vi "校准任务流程.vi"(9 "校准任务":T1[](array[typedef]), 10 "精度":dbl=4.0, 11 "模型":enum32{"线性", "多项式", "折线"}(ring)) -> ()   [LabVIEW 2016]
uses:
  <userlib>/_OpenG.lib/array/array.llb/Remove Duplicates from 1D Array (U16)__ogtk.vi
panel:
  out "元素":T1
  out "执行列表":T2(ring)
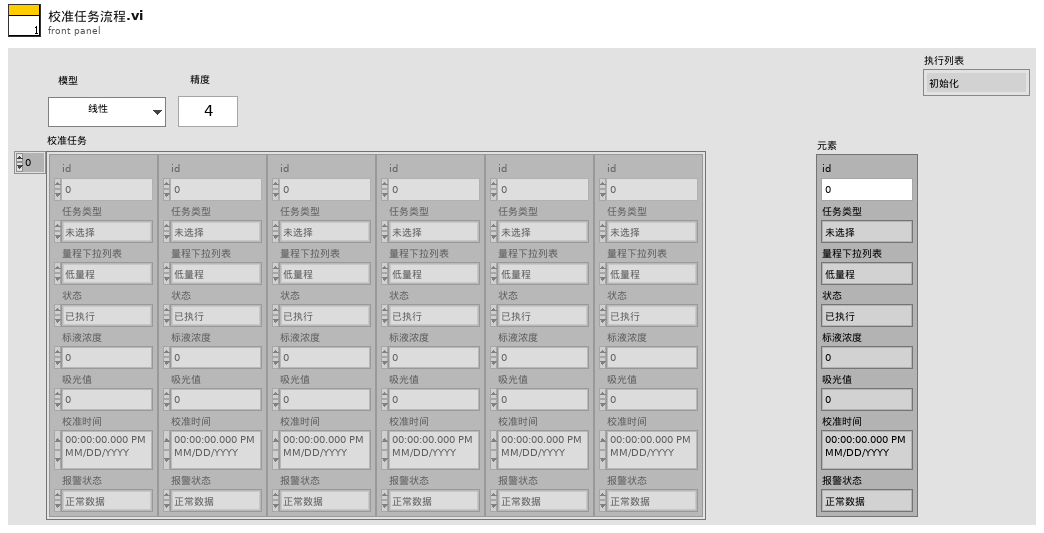
[diagram p1: front panel]
types:
  T1 = typedef "校准任务.ctl" = cluster{"id":u16, "任务类型":enum16{"未选择", "空白校准", "标样校准", "标样核查", "零点核查", "跨度核查"}, "量程下拉列表":enum16{"低量程", "高量程"}, "状态":enum16{"已执行", "待执行", "执行中", "停止"}, "标液浓度":dbl, "吸光值":dbl, "校准时间":timestamp, "报警状态":enum16{"正常数据", "报警数据"}}
  T2 = enum16{"初始化", "解析数据", "判断任务类型", "执行测试任务", "等待测试任务完成", "获取测试数据", "任务结束判定", "计算公式", "结束"}
  T3 = cluster{"时间标识":timestamp, "设备":string, "日志信息":string, "流程参数":string}
  T4 = cluster{"站号":u16, "量程切换":enum32{"H", "L", "AUTO"}, "控制命令":u16, "模式设置":enum16{"待机", "连续模式", "周期模式", "定点模式", "受控模式", "手动模式"}, "测量间隔":u16}
  T5 = cluster{"标液浓度1":dbl, "测量吸光度1":dbl, "样品1启用":bool, "标液浓度2":dbl, "测量吸光度2":dbl, "样品2启用":bool, "标液浓度3":dbl, "测量吸光度3":dbl, "样品3启用":bool, "标液浓度4":dbl, "测量吸光度4":dbl, "样品4启用":bool, "标液浓度5":dbl, "测量吸光度5":dbl, "样品5启用":bool, "模型":enum32{"线性", "多项式", "折线"}, "精度":dbl, "XY图":cluster{"X Values":dbl[], "Y Values":dbl[]}[], "拟合公式":string, "r^2":dbl, "标样一校准时间":timestamp, "标样二校准时间":timestamp, "标样三校准时间":timestamp, "标样四校准时间":timestamp, "标样五校准时间":timestamp, "二次方程":cluster{"x^2":dbl, "K":dbl, "B":dbl}, "标定时间":timestamp, "拟合公式 2":string, "r^2 2":dbl}
  T6 = enum16{"", "水样测量", "标样核查", "零点核查", "跨度核查", "空白测试", "平行样测试", "加标回收", "空白校准", "标样校准"}
  T7 = typedef "报警信息字段定义.ctl" = cluster{"时间":timestamp, "参数":string, "元器件":string, "故障现象":string, "故障分析":string, "state":string, "code":string, "platform_alarm_code":string}
  T8 = cluster{"测量精度":u16, "消解温度":u16, "消解时长":u16, "量程下限":sgl, "量程上限":sgl, "曲线斜率K":sgl, "曲线斜率B":sgl, "标定日期":timestamp, "标液1浓度":sgl, "标液1测量过程值":sgl, "标液2浓度":sgl, "标液2测量过程值":sgl, "标液3浓度":sgl, "标液3测量过程值":sgl, "标液4浓度":sgl, "标液4测量过程值":sgl, "标液5浓度":sgl, "标液5测量过程值":sgl, "线性相关系数":sgl, "试剂余量":u32, "测量滴定值或吸光度":sgl, "标样2校准时间":timestamp, "检出限值":sgl, "校准系数":sgl, "设备系列号":string, "显色温度":u16, "显色时间":u16, "试剂余量1":u16, "试剂余量2":u16, "试剂余量3":u16, "试剂余量4":u16, "试剂余量5":u16, "试剂余量6":u16, "试剂余量7":u16, "试剂余量8":u16, "试剂余量9":u16, "试剂余量10":u16, "当前量程低位":sgl, "当前量程高位":sgl}
  T9 = cluster{"因子编码":u32, "单位":u16, "标样2参考值":sgl, "水样数据时间":timestamp, "水样实测值":sgl, "水样数据标识":string, "标样2数据时间":timestamp, "标样2实测值":sgl, "标样2数据标识":string, "空白数据时间":timestamp, "空白实测值":sgl, "空白数据标识":string, "零点核查数据时间":timestamp, "零点核查实测值":sgl, "零点核查数据标识":string, "跨度核查数据时间":timestamp, "跨度核查实测值":sgl, "跨度核查数据标识":string, "加标回收数据时间":timestamp, "加标回收实测值":sgl, "加标回收数据标识":string, "平行样数据时间":timestamp, "平行样实测值":sgl, "平行样数据标识":string, "标样1参考值":sgl, "标样1数据时间":timestamp, "标样1实测值":sgl, "标样1数据标识":string, "标样核查数据时间":timestamp, "标样核查实测值":sgl, "标样核查数据标识":string}
  T10 = cluster{"系统时间":timestamp, "工作状态":u16, "测量模式":enum16{"待机", "连续模式", "周期模式", "定点模式", "受控模式", "手动模式"}, "告警代码":u16, "故障代码":u16, "日志代码":u16, "软件版本":u16, "测量间隔":u16, "消解实时温度":dbl, "校准间隔（天）":u16, "校准间隔（时）":u16, "周期测量时间（23_16）":u16, "周期测量时间（15_0）":u16, "清洗周期（次数）":u16, "运行模式":u16, "自动校准状态":u16, "自动清洗状态":u16}
  T11 = enum16{"未选择", "空白校准", "标样校准", "标样核查", "零点核查", "跨度核查"}
  T12 = cluster{"标液浓度1":dbl, "测量吸光度1":dbl, "样品1启用":bool, "标液浓度2":dbl, "测量吸光度2":dbl, "样品2启用":bool, "标液浓度3":dbl, "测量吸光度3":dbl, "样品3启用":bool, "标液浓度4":dbl, "测量吸光度4":dbl, "样品4启用":bool, "标液浓度5":dbl, "测量吸光度5":dbl, "样品5启用":bool, "模型":enum32{"线性", "多项式", "折线"}, "精度":dbl, "XY图":cluster{"X Values":dbl[], "Y Values":dbl[]}[], "拟合公式":string, "r^2":dbl, "标样一校准时间":timestamp, "标样二校准时间":timestamp, "标样三校准时间":timestamp, "标样四校准时间":timestamp, "标样五校准时间":timestamp, "二次方程":cluster{"c":dbl, "x":dbl, "x^2":dbl}, "标定时间":timestamp, "拟合公式 2":string, "r^2 2":dbl}
  T13 = cluster{"标液浓度1":dbl, "测量吸光度1":dbl, "样品1启用":bool, "标液浓度2":dbl, "测量吸光度2":dbl, "样品2启用":bool, "标液浓度3":dbl, "测量吸光度3":dbl, "样品3启用":bool, "标液浓度4":dbl, "测量吸光度4":dbl, "样品4启用":bool, "标液浓度5":dbl, "测量吸光度5":dbl, "样品5启用":bool, "模型":enum32{"线性", "多项式", "折线"}, "精度":dbl, "XY图":cluster{"X Values":dbl[], "Y Values":dbl[]}[], "拟合公式":string, "r^2":dbl, "标样一校准时间":timestamp, "标样二校准时间":timestamp, "标样三校准时间":timestamp, "标样四校准时间":timestamp, "标样五校准时间":timestamp, "二次方程":cluster{"c":dbl, "x":dbl, "x^2":dbl}, "标定时间":timestamp, "拟合公式 2":string, "r^2 2":dbl}[][]
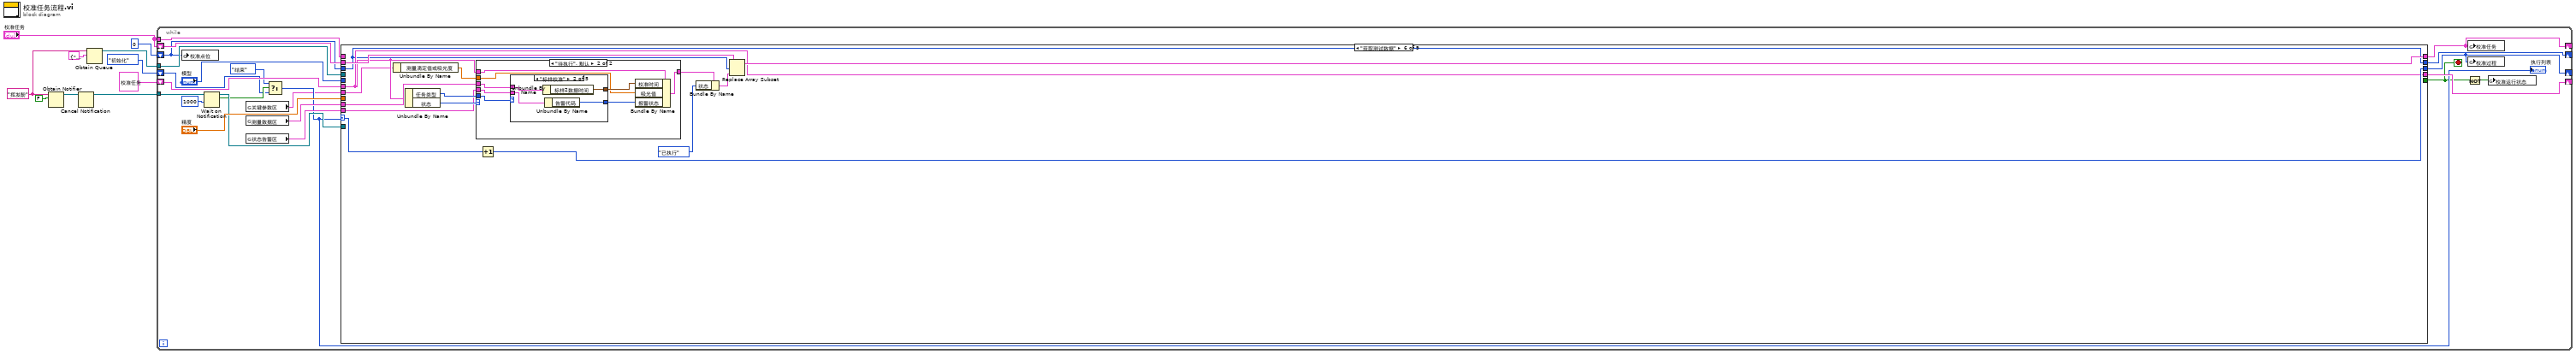
[diagram p0: block diagram]
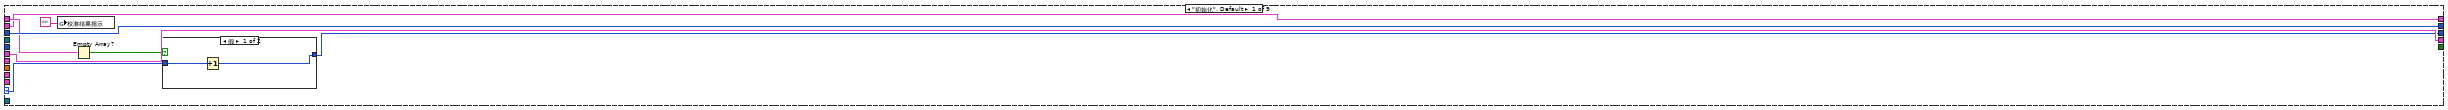
[diagram p2: hidden frame]
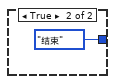
[diagram p3: hidden frame]
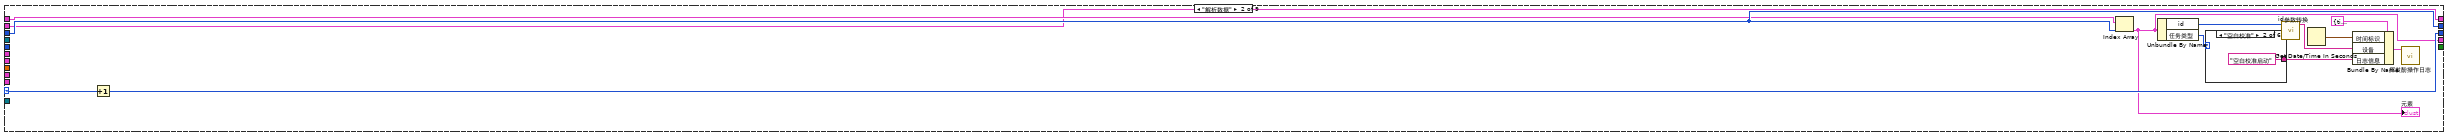
[diagram p4: hidden frame]
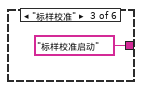
[diagram p6: hidden frame]
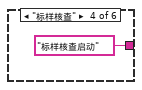
[diagram p7: hidden frame]
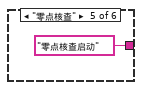
[diagram p8: hidden frame]
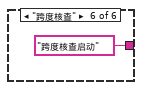
[diagram p9: hidden frame]
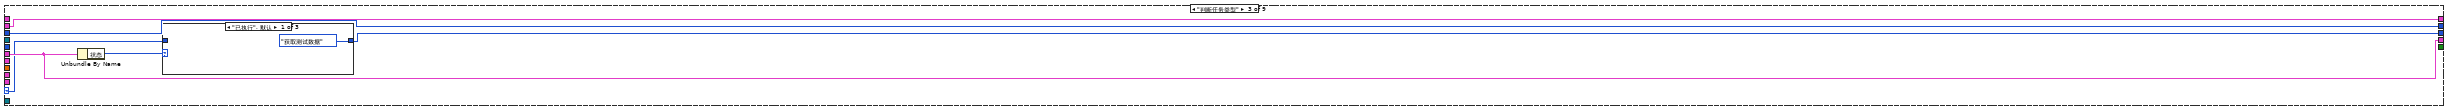
[diagram p10: hidden frame]
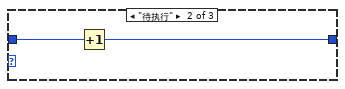
[diagram p11: hidden frame]
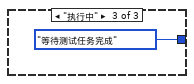
[diagram p12: hidden frame]
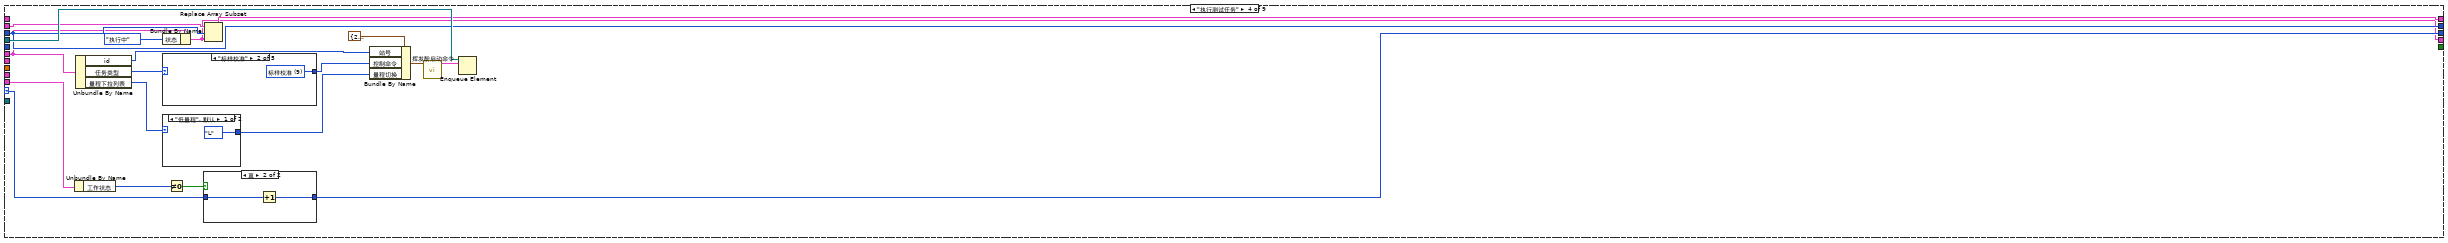
[diagram p13: hidden frame]
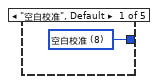
[diagram p15: hidden frame]
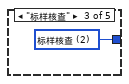
[diagram p16: hidden frame]
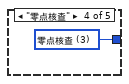
[diagram p17: hidden frame]
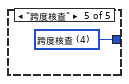
[diagram p18: hidden frame]
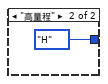
[diagram p19: hidden frame]
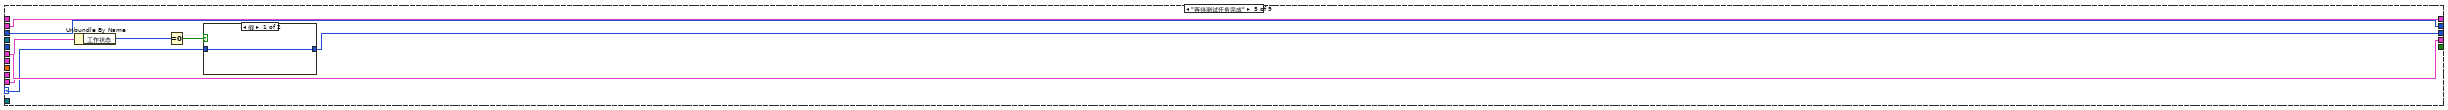
[diagram p20: hidden frame]
diagram:
  w2 = "挥发酚" ("名称（未命名）")
  n1 = Obtain Notifier(name (unnamed)=w2, notification data type=FALSE) -> (notifier out=w5:refnum<notifier>)  [unwired: 2 in, 2 out]
  n2 = Cancel Notification(0:w5) -> (8:w4:refnum<notifier>)  [unwired: 1 in, 2 out]
  n3 = Obtain Queue(name (unnamed)=w2, element data type=cluster{"命令":string, "data":variant} {"命令"="", "data"=variant}) -> (queue out=w6:refnum<queue>)  [unwired: 3 in, 2 out]
  n4 = while {
    shift-right: [w13] -> _
    shift-left: 0 -> [w15]
    shift-right: [w33] -> _
    shift-left: T1 {"id"=0, "任务类型"=enum."未选择", "量程下拉列表"=enum."低量程", "状态"=enum."待执行", "标液浓度"=0.0, "吸光值"=0.0, "校准时间"=timestamp(0 s since 1904-01-01), "报警状态"=enum."正常数据"} ("校准任务") -> [w32]
    shift-right: [w12] -> _
    shift-left: T2."初始化" ("执行列表") -> [w21]
    tunnel: w6 -> [w31]
    tunnel: w4 -> [w30]
    tunnel: "校准任务" -> [w27]
    shift-right: [w14] -> _
    shift-left: "校准任务" -> [w26]
    stop <- w16 stop-if-true
    n5 = global write "VAR挥发酚全局变量.vi" "校准点位"(w15) -> ()
    n6 = Wait on Notification(notifier=w30, timeout in ms (-1)=1000 ("超时毫秒(-1)")) -> (notifier out=w23:refnum<notifier>, notification=w22:bool)  [unwired: 2 in, 2 out]
    n7 = global read "VAR挥发酚全局变量.vi" "关键参数区"() -> (w11:T8)
    n8 = global read "VAR挥发酚全局变量.vi" "测量数据区"() -> (w28:T9)
    n9 = global read "VAR挥发酚全局变量.vi" "状态告警区"() -> (w29:T10)
    n10 = Select(t=T2."结束", s=w22, f=w21) -> (s? t:f=w20:T2)
    "执行列表" <- w20
    n11 = case shown="\"获取测试数据\"" w20 {
      selector: w20 -> [w39 w56 w65 w83 w106 w126 w164 w178 w372]
      tunnel: w15 -> [w40 w57 w67 w79 w109 w117 w165 w176 w370]
      tunnel: [w41 w48 w68 w76 w110 w121 w166 w175 w371] -> w33
      tunnel: w32 -> [w41 _ w68 w78 w110 w121 w166 w175 w371]
      tunnel: [w40 w57 w67 w79 w109 w117 w161 w176 w370] -> w13
      tunnel: [_ _ _ _ _ _ _ _ TRUE] -> w16
      tunnel: [w38 w55 w64 w82 w104 w125 w163 w177 w372] -> w12
      tunnel: w31 -> [_ _ _ w91 _ _ _ _ w367]
      tunnel: w23 -> [_ _ _ _ _ _ _ _ w366]
      tunnel: w29 -> [_ _ _ w86 w108 w116 _ _ _]
      tunnel: w28 -> [_ _ _ _ _ w128 _ _ _]
      tunnel: w27 -> [w36 w54 _ _ _ _ w162 _ _]
      tunnel: [w35 w53 w63 w80 w103 w123 w158 w174 w368] -> w14
      tunnel: w26 -> [w35 w53 w63 w81 w103 w122 w158 w174 w368]
      tunnel: "模型" -> [_ _ _ _ _ _ _ w173 _]
      tunnel: "精度" -> [_ _ _ _ _ _ _ w172 _]
      tunnel: w11 -> [_ _ _ _ _ w115 _ _ _]
      frame "初始化", Default {
        n12 = global write "VAR挥发酚全局变量.vi" "校准结果指示"("") -> ()
        n13 = Empty Array?(array=w36) -> (empty?=w34:bool)
        n14 = case shown="假" w34 {
          tunnel: w39 -> [w43 _]
          tunnel: [w42 T2."结束"] -> w38
          frame False {
            n15 = Increment(x=w43) -> (x+1=w42:T2)
          }
          frame True {
          }
        }
      }
      frame "解析数据" {
        n16 = Increment(x=w56) -> (x+1=w55:T2)
        n17 = Index Array(array=w54, index=w57) -> (element=w48:T1)
        "元素" <- w48
        n18 = Unbundle By Name(w48) -> ("id"=w47:u16, "任务类型"=w46:T11)
        n19 = case shown="\"空白校准\"" w46 {
          tunnel: [_ "空白校准启动" "标样校准启动" "标样核查启动" "零点核查启动" "跨度核查启动"] -> w45
          frame "未选择", Default {
          }
          frame "空白校准" {
          }
          frame "标样校准" {
          }
          frame "标样核查" {
          }
          frame "零点核查" {
          }
          frame "跨度核查" {
          }
        }
        n20 = call "id参数转换.vi"("id"=w47) -> ("table输出"=w49:string)  [unwired: 10 in]
        n21 = Get Date/Time In Seconds() -> (seconds since 1Jan1904=w52:timestamp)
        n22 = Bundle By Name(cluster=T3 {"时间标识"=timestamp(0 s since 1904-01-01), "设备"="", "日志信息"="", "流程参数"=""} ("data in"), "时间标识"=w52, "设备"=w49, "日志信息"=w45) -> (w51:T3)
        n23 = call "挥发酚操作日志.vi"("data in"=w51) -> ()  [unwired: 11 in]
      }
      frame "判断任务类型" {
        n24 = Unbundle By Name(w68) -> ("状态"=w66:enum16{"已执行", "待执行", "执行中", "停止"})
        n25 = case shown="\"已执行\", 默认" w66 {
          tunnel: w65 -> [_ w71 _]
          tunnel: [T2."获取测试数据" w70 T2."等待测试任务完成"] -> w64
          frame "已执行", Default {
          }
          frame "待执行" {
            n26 = Increment(x=w71) -> (x+1=w70:T2)
          }
          frame "执行中" {
          }
        }
      }
      frame "执行测试任务" {
        n27 = Unbundle By Name(w86) -> ("工作状态"=w85:u16)
        n28 = Unbundle By Name(w78) -> ("id"=w90:u16, "任务类型"=w89:T11, "量程下拉列表"=w88:enum16{"低量程", "高量程"})
        n29 = Bundle By Name(cluster=w78, "状态"=enum16{"已执行", "待执行", "执行中", "停止"}."执行中") -> (w76:T1)
        n30 = case shown="\"标样校准\"" w89 {
          tunnel: [w96 w97 w98 w99 w100] -> w73
          frame "空白校准", Default {
            w96 = u16 8 items=["启动测量"=1, "标样核查"=2, "零点核查"=3, "跨度核查"=4, "空白测试"=5, "平行样测试"=6, "加标回收"=7, "空白校准"=8, "标样校准"=9, "初始化（清洗）"=10, "停止测试"=11, "仪器重启"=12, "校时"=13, "模式设置"=14, "测量间隔设置"=15, "调试"=22, "填充管路"=30, "清洗管路"=31, "清洗反应杯"=32] ("控制命令")
          }
          frame "标样校准" {
            w97 = u16 9 items=["启动测量"=1, "标样核查"=2, "零点核查"=3, "跨度核查"=4, "空白测试"=5, "平行样测试"=6, "加标回收"=7, "空白校准"=8, "标样校准"=9, "初始化（清洗）"=10, "停止测试"=11, "仪器重启"=12, "校时"=13, "模式设置"=14, "测量间隔设置"=15, "调试"=22, "填充管路"=30, "清洗管路"=31, "清洗反应杯"=32] ("控制命令")
          }
          frame "标样核查" {
            w98 = u16 2 items=["启动测量"=1, "标样核查"=2, "零点核查"=3, "跨度核查"=4, "空白测试"=5, "平行样测试"=6, "加标回收"=7, "空白校准"=8, "标样校准"=9, "初始化（清洗）"=10, "停止测试"=11, "仪器重启"=12, "校时"=13, "模式设置"=14, "测量间隔设置"=15, "调试"=22, "填充管路"=30, "清洗管路"=31, "清洗反应杯"=32] ("控制命令")
          }
          frame "零点核查" {
            w99 = u16 3 items=["启动测量"=1, "标样核查"=2, "零点核查"=3, "跨度核查"=4, "空白测试"=5, "平行样测试"=6, "加标回收"=7, "空白校准"=8, "标样校准"=9, "初始化（清洗）"=10, "停止测试"=11, "仪器重启"=12, "校时"=13, "模式设置"=14, "测量间隔设置"=15, "调试"=22, "填充管路"=30, "清洗管路"=31, "清洗反应杯"=32] ("控制命令")
          }
          frame "跨度核查" {
            w100 = u16 4 items=["启动测量"=1, "标样核查"=2, "零点核查"=3, "跨度核查"=4, "空白测试"=5, "平行样测试"=6, "加标回收"=7, "空白校准"=8, "标样校准"=9, "初始化（清洗）"=10, "停止测试"=11, "仪器重启"=12, "校时"=13, "模式设置"=14, "测量间隔设置"=15, "调试"=22, "填充管路"=30, "清洗管路"=31, "清洗反应杯"=32] ("控制命令")
          }
        }
        n31 = case shown="\"低量程\", 默认" w88 {
          tunnel: [enum32{"H", "L", "AUTO"}."L" ("量程切换") enum32{"H", "L", "AUTO"}."H" ("量程切换")] -> w87
          frame "低量程", Default {
          }
          frame "高量程" {
          }
        }
        n32 = Not Equal To 0?(x=w85) -> (x != 0?=w84:bool)
        n33 = case shown="真" w84 {
          tunnel: w83 -> [w93 w95]
          tunnel: [w93 w94] -> w82
          frame False {
          }
          frame True {
            n34 = Increment(x=w95) -> (x+1=w94:T2)
          }
        }
        n35 = Replace Array Subset(array=w81, new element=w76, index=w79) -> (w80:T1[])
        n36 = Bundle By Name(cluster=T4 {"站号"=21, "量程切换"=enum."AUTO", "控制命令"=0, "模式设置"=enum."待机", "测量间隔"=0} ("参数"), "站号"=w90, "控制命令"=w73, "量程切换"=w87) -> (w74:T4)
        n37 = call "挥发酚启动命令.vi"("参数"=w74) -> ("启动命令"=w92:cluster{"命令":string, "data":variant})  [unwired: 10 in]
        n38 = Enqueue Element(queue=w91, element=w92) -> ()  [unwired: 2 in, 3 out]
      }
      frame "等待测试任务完成" {
        n39 = Unbundle By Name(w108) -> ("工作状态"=w107:u16)
        n40 = Equal To 0?(x=w107) -> (x = 0?=w105:bool)
        n41 = case shown="假" w105 {
          tunnel: w106 -> [w111 w113]
          tunnel: [w111 w112] -> w104
          frame False {
          }
          frame True {
            n42 = Increment(x=w113) -> (x+1=w112:T2)
          }
        }
      }
      frame "获取测试数据" {
        n43 = Unbundle By Name(w115) -> ("测量滴定值或吸光度"=w114:sgl)
        n44 = Unbundle By Name(w121) -> ("任务类型"=w127:T11, "状态"=w120:enum16{"已执行", "待执行", "执行中", "停止"})
        n45 = case shown="\"待执行\", 默认" w120 {
          tunnel: w128 -> [_ w137]
          tunnel: w127 -> [_ w136]
          tunnel: [w129 w134] -> w124
          tunnel: w121 -> [w129 w133]
          tunnel: w116 -> [_ w132]
          tunnel: w114 -> [_ w130]
          frame "已执行" {
          }
          frame "待执行", Default {
            n46 = case shown="\"标样校准\"" w136 {
              tunnel: w137 -> [w141 w145 w149 w153 w157]
              tunnel: [w140 w144 w148 w152 w156] -> w135
              tunnel: w132 -> [w139 w143 w147 w151 w155]
              tunnel: [w138 w142 w146 w150 w154] -> w131
              frame "空白校准", Default {
                n47 = Unbundle By Name(w141) -> ("空白数据时间"=w140:timestamp)
                n48 = Unbundle By Name(w139) -> ("告警代码"=w138:u16)
              }
              frame "标样校准" {
                n49 = Unbundle By Name(w145) -> ("标样2数据时间"=w144:timestamp)
                n50 = Unbundle By Name(w143) -> ("告警代码"=w142:u16)
              }
              frame "标样核查" {
                n51 = Unbundle By Name(w149) -> ("标样2数据时间"=w148:timestamp)
                n52 = Unbundle By Name(w147) -> ("告警代码"=w146:u16)
              }
              frame "零点核查" {
                n53 = Unbundle By Name(w153) -> ("零点核查数据时间"=w152:timestamp)
                n54 = Unbundle By Name(w151) -> ("告警代码"=w150:u16)
              }
              frame "跨度核查" {
                n55 = Unbundle By Name(w157) -> ("跨度核查数据时间"=w156:timestamp)
                n56 = Unbundle By Name(w155) -> ("告警代码"=w154:u16)
              }
            }
            n57 = Bundle By Name(cluster=w133, "校准时间"=w135, "吸光值"=w130, "报警状态"=w131) -> (w134:T1)
          }
        }
        n58 = Increment(x=w126) -> (x+1=w125:T2)
        n59 = Bundle By Name(cluster=w124, "状态"=enum16{"已执行", "待执行", "执行中", "停止"}."已执行") -> (w118:T1)
        n60 = Replace Array Subset(array=w122, new element=w118, index=w117) -> (w123:T1[])
      }
      frame "任务结束判定" {
        n61 = Array Size(array=w162) -> (size(s)=w160:i32)
        n62 = Increment(x=w165) -> (x+1=w161:i32)
        n63 = Greater Or Equal?(x=w161, y=w160) -> (x >= y?=w159:bool)
        n64 = case shown="假" w159 {
          tunnel: w164 -> [_ w170]
          tunnel: [T2."解析数据" w169] -> w163
          frame False {
            n65 = Wait (ms)(milliseconds to wait=u32 3000 ("等待时间（毫秒）")) -> ()  [unwired: 1 out]
          }
          frame True {
            n66 = Increment(x=w170) -> (x+1=w169:T2)
          }
        }
      }
      frame "计算公式" {
        n67 = flat-sequence {
          tunnel: w178 -> [w185]
          tunnel: w174 -> [w181]
          tunnel: w173 -> [w180]
          tunnel: w172 -> [w179]
          tunnel: [w184] -> w171
          tunnel: [w365] -> w177
          tunnel: w171 -> [w365]
          frame #0 {
            n68 = for {
              tunnel: w181 -> [w364] mode=indexing
              tunnel: [w363] -> w183 mode=indexing
              n69 = Unbundle By Name(w364) -> ("id"=w363:u16)
            }
            n70 = Increment(x=w185) -> (x+1=w184:T2)
            n71 = call-poly <userlib>:"Remove Duplicates from 1D Array__ogtk.vi"("Input Array"=w183) -> ("Output Array"=w182:u16[])  [unwired: 1 out]
            n72 = for {
              tunnel: w182 -> [w198] mode=indexing
              tunnel: w181 -> [w200]
              tunnel: w180 -> [w197]
              tunnel: w179 -> [w196]
              n73 = for {
                tunnel: w200 -> [w360] mode=indexing
                tunnel: w198 -> [w362]
                tunnel: [w360] -> w199 mode=indexing if=w361
                n74 = Unbundle By Name(w360) -> ("id"=w359:u16)
                n75 = Equal?(x=w359, y=w362) -> (x = y?=w361:bool)
              }
              n76 = flat-sequence {
                tunnel: w199 -> [w213]
                tunnel: w198 -> [w208]
                tunnel: w197 -> [w212]
                tunnel: w196 -> [w211]
                tunnel: T5 {"标液浓度1"=0.0, "测量吸光度1"=0.0, "样品1启用"=FALSE, "标液浓度2"=0.0, "测量吸光度2"=0.0, "样品2启用"=FALSE, "标液浓度3"=0.0, "测量吸光度3"=0.0, "样品3启用"=FALSE, "标液浓度4"=0.0, "测量吸光度4"=0.0, "样品4启用"=FALSE, "标液浓度5"=0.0, "测量吸光度5"=0.0, "样品5启用"=FALSE, "模型"=enum."线性", "精度"=4.0, "XY图"=[], "拟合公式"="", "r^2"=0.0, "标样一校准时间"=timestamp(0 s since 1904-01-01), "标样二校准时间"=timestamp(0 s since 1904-01-01), "标样三校准时间"=timestamp(0 s since 1904-01-01), "标样四校准时间"=timestamp(0 s since 1904-01-01), "标样五校准时间"=timestamp(0 s since 1904-01-01), "二次方程"={"x^2"=0.0, "K"=0.0, "B"=0.0}, "标定时间"=timestamp(0 s since 1904-01-01), "拟合公式 2"="", "r^2 2"=0.0} ("曲线模型") -> [w210]
                tunnel: [w209] -> w195
                tunnel: [w208] -> w194
                tunnel: [w207] -> w193
                tunnel: [w206] -> w191
                tunnel: cluster{"x^2":dbl, "K":dbl, "B":dbl} {"x^2"=0.0, "K"=0.0, "B"=0.0} ("二次方程 2") -> [w205]
                tunnel: [w204] -> w190
                tunnel: 0.0 ("公式切换阈值滴定数(0~9999)") -> [w203]
                tunnel: [w202] -> w188
                tunnel: TRUE -> [w201]
                tunnel: w195 -> [w287]
                tunnel: w194 -> [w289]
                tunnel: w193 -> [w288]
                tunnel: w191 -> [w285]
                tunnel: w190 -> [w284]
                tunnel: w188 -> [w279]
                frame #0 {
                  n77 = for {
                    tunnel: w213 -> [w235] mode=indexing
                    tunnel: w208 -> [_]
                    tunnel: w212 -> [w232]
                    tunnel: w211 -> [w231]
                    shift-right: [w223] -> w209
                    shift-left: w210 -> [w230]
                    tunnel: [w221] -> w207
                    shift-right: [w220] -> w206
                    shift-left: w205 -> [_]
                    shift-right: [w219] -> w204
                    shift-left: w203 -> [_]
                    shift-right: [w216] -> w202
                    shift-left: w201 -> [w214]
                    n78 = Unbundle By Name(w235) -> ("标液浓度"=w234:dbl, "吸光值"=w233:dbl, "任务类型"=w222:T11, "量程下拉列表"=w221:enum16{"低量程", "高量程"}, "校准时间"=w229:timestamp, "报警状态"=w217:enum16{"正常数据", "报警数据"})
                    n79 = Greater Than 0?(x=w217) -> (x > 0?=w215:bool)
                    n80 = case shown="\"空白校准\"" w222 {
                      tunnel: w234 -> [_ w246 w254 w262 w270 w278]
                      tunnel: w233 -> [_ w245 w247 w261 w269 w277]
                      tunnel: w232 -> [_ w244 w253 w260 w268 w276]
                      tunnel: w231 -> [_ w243 w252 w259 w267 w275]
                      tunnel: w230 -> [w238 w241 w250 w257 w265 w273]
                      tunnel: [w238 w239 w249 w256 w264 w272] -> w228
                      tunnel: w229 -> [_ w240 w248 w255 w263 w271]
                      frame "未选择", Default {
                        (unwired) T6."" ("测量模式")
                      }
                      frame "空白校准" {
                        n81 = Bundle By Name(cluster=w241, "标液浓度1"=w246, "测量吸光度1"=w245, "模型"=w244, "精度"=w243, "样品1启用"=TRUE, "标样一校准时间"=w240) -> (w239:T5)
                      }
                      frame "标样校准" {
                        (unwired) T6."标样校准" ("测量模式")
                        n82 = Bundle By Name(cluster=w250, "标液浓度2"=w254, "测量吸光度2"=w247, "模型"=w253, "精度"=w252, "样品2启用"=TRUE ("样品1启用"), "标样二校准时间"=w248) -> (w249:T5)
                      }
                      frame "标样核查" {
                        (unwired) T6."标样核查" ("测量模式")
                        n83 = Bundle By Name(cluster=w257, "标液浓度3"=w262, "测量吸光度3"=w261, "模型"=w260, "精度"=w259, "样品3启用"=TRUE ("样品1启用"), "标样三校准时间"=w255) -> (w256:T5)
                      }
                      frame "零点核查" {
                        (unwired) T6."零点核查" ("测量模式")
                        n84 = Bundle By Name(cluster=w265, "标液浓度4"=w270, "测量吸光度4"=w269, "模型"=w268, "精度"=w267, "样品4启用"=TRUE ("样品1启用"), "标样四校准时间"=w263) -> (w264:T5)
                      }
                      frame "跨度核查" {
                        (unwired) T6."跨度核查" ("测量模式")
                        n85 = Bundle By Name(cluster=w273, "标液浓度5"=w278, "测量吸光度5"=w277, "模型"=w276, "精度"=w275, "样品5启用"=TRUE ("样品1启用"), "标样五校准时间"=w271) -> (w272:T5)
                      }
                    }
                    n86 = case shown="假" w215 {
                      tunnel: [w236 FALSE] -> w216
                      tunnel: w214 -> [w236 _]
                      frame False {
                      }
                      frame True {
                      }
                    }
                    n87 = call "曲线模型计算.vi"("曲线模型"=w228) -> ("公式切换阈值滴定数(0~9999)"=w219:dbl, "二次方程 2"=w220:cluster{"x^2":dbl, "K":dbl, "B":dbl}, "输出簇"=w224:T12)  [unwired: 8 in]
                    n88 = global read "校准数据全局变量.vi" "CODMn曲线模型"() -> (w227:T13)
                    n89 = Get Date/Time In Seconds() -> (seconds since 1Jan1904=w225:timestamp)
                    n90 = Bundle By Name(cluster=w224, "标定时间"=w225) -> (w223:T12)
                    n91 = Replace Array Subset(array=w227, new element=w223, index (row)=T6."水样测量" ("测量模式"), index (col)=w221) -> (w226:T13)
                    n92 = global write "校准数据全局变量.vi" "CODMn曲线模型"(w226) -> ()
                  }
                }
                frame #1 {
                  n93 = Unbundle By Name(w287) -> ("r^2"=w282:dbl, "r^2 2"=w281:dbl, "二次方程"=w290:cluster{"x^2":dbl, "K":dbl, "B":dbl}, "模型"=w283:enum32{"线性", "多项式", "折线"})
                  n94 = case shown="\"线性\", 默认" w283 {
                    tunnel: w282 -> [w295 w299]
                    tunnel: w281 -> [_ w300]
                    tunnel: [w292 w301] -> w280
                    tunnel: w279 -> [w291 w297]
                    frame "线性", Default {
                      n95 = global read "挥发酚断电保存全局变量.vi" "校准条件"() -> (w296:cluster{"线性相关系数":dbl})
                      n96 = Unbundle By Name(w296) -> ("线性相关系数"=w294:dbl)
                      n97 = Greater Or Equal?(x=w295, y=w294) -> (x >= y?=w293:bool)
                      n98 = And(x=w291, y=w293) -> (x .and. y?=w292:bool)
                    }
                    frame "折线" {
                      n99 = global read "挥发酚断电保存全局变量.vi" "校准条件"() -> (w304:cluster{"线性相关系数":dbl})
                      n100 = Unbundle By Name(w304) -> ("线性相关系数"=w298:dbl)
                      n101 = Greater Or Equal?(x=w299, y=w298) -> (x >= y?=w303:bool)
                      n102 = Greater Or Equal?(x=w300, y=w298) -> (x >= y?=w302:bool)
                      n103 = Compound Arithmetic op=AND ("复合运算")(w303, w302, w297) -> (w301:bool)
                    }
                  }
                  n104 = case shown="真" w280 {
                    tunnel: w290 -> [_ w329]
                    tunnel: w289 -> [w310 _]
                    tunnel: w288 -> [_ w318]
                    tunnel: w287 -> [_ w328]
                    tunnel: [w305 w327] -> w286
                    tunnel: w285 -> [_ w326]
                    tunnel: w284 -> [_ w317]
                    tunnel: w279 -> [w307 _]
                    frame False {
                      n105 = case shown="假" w307 {
                        tunnel: ["有故障数据" ("格式字符串") "校准条件未满足" ("格式字符串")] -> w306
                        frame False {
                        }
                        frame True {
                        }
                      }
                      n106 = call "id参数转换.vi"("id"=w310) -> ("table输出"=w309:string)  [unwired: 10 in]
                      n107 = Format Into String(format string="校准失败，%s" ("格式字符串"), w306) -> (resulting string=w305:string)  [unwired: 2 in, 1 out]
                      n108 = Get Date/Time In Seconds() -> (seconds since 1Jan1904=w313:timestamp)
                      n109 = Bundle By Name(cluster=T3 {"时间标识"=timestamp(0 s since 1904-01-01), "设备"="", "日志信息"="", "流程参数"=""} ("data in"), "时间标识"=w313, "设备"=w309, "日志信息"=w305) -> (w312:T3)
                      n110 = call "挥发酚操作日志.vi"("data in"=w312) -> ()  [unwired: 11 in]
                    }
                    frame True {
                      n111 = Unbundle By Name(w326) -> ("x^2"=w322:dbl, "K"=w321:dbl, "B"=w320:dbl)
                      n112 = Unbundle By Name(w329) -> ("x^2"=w331:dbl, "K"=w332:dbl, "B"=w333:dbl)
                      n113 = Bundle By Name(cluster=cluster{"X^2":dbl, "X":dbl, "b":dbl} {"X^2"=0.0, "X"=0.0, "b"=0.0} ("公式"), "X^2"=w322, "X"=w321, "b"=w320) -> (w319:cluster{"X^2":dbl, "X":dbl, "b":dbl})
                      n114 = Bundle By Name(cluster=cluster{"X^2":dbl, "X":dbl, "b":dbl} {"X^2"=0.0, "X"=0.0, "b"=0.0} ("公式"), "X^2"=w331, "X"=w332, "b"=w333) -> (w324:cluster{"X^2":dbl, "X":dbl, "b":dbl})
                      n115 = for {
                        N: 7 -> [_]
                        tunnel: w324 -> [w344]
                        tunnel: [w342] -> w316
                        tunnel: w319 -> [w341]
                        tunnel: w317 -> [w340]
                        tunnel: w318 -> [w338]
                        i -> [w335]
                        w339 = enum16{"CODMn"}."CODMn" ("测量参数")
                        n116 = case shown="\"高量程\"" w338 {
                          tunnel: [enum16{"低量程1", "低量程2", "高量程1", "高量程2"}."低量程1" ("量程") enum16{"低量程1", "低量程2", "高量程1", "高量程2"}."高量程1" ("量程")] -> w337
                          tunnel: [enum16{"低量程1", "低量程2", "高量程1", "高量程2"}."低量程2" ("量程") enum16{"低量程1", "低量程2", "高量程1", "高量程2"}."高量程2" ("量程")] -> w336
                          frame "低量程", Default {
                          }
                          frame "高量程" {
                          }
                        }
                        n117 = Increment(x=w335) -> (x+1=w334:i32)
                        n118 = call "公式写入.vi"("临界滴定数"=w340, "公式"=w344, "error in (no error)"=errorcluster {"status"=FALSE, "code"=0, "source"=""} ("error out"), "量程"=w337, "测量模式"=w334, "测量参数"=w339) -> ("error out"=w343:errorcluster)  [unwired: 5 in]
                        n119 = call "公式写入.vi"("临界滴定数"=w340, "公式"=w341, "error in (no error)"=w343, "量程"=w336, "测量模式"=w334, "测量参数"=w339) -> ("error out"=w342:errorcluster)  [unwired: 5 in]
                      }
                      n120 = case shown="错误" w316 {
                        tunnel: w318 -> [w353 _]
                        tunnel: w328 -> [w351 _]
                        tunnel: ["校准成功" w356] -> w327
                        frame No Error {
                          n121 = call "校准记录.vi"("曲线模型"=w351, "量程"=w353, "测量模式"="所有测量模式") -> ()  [unwired: 8 in, 1 out]
                        }
                        frame Error {
                          w356 = "校准失败，公式写入异常"
                          n122 = Get Date/Time In Seconds() -> (seconds since 1Jan1904=w357:timestamp)
                          n123 = Bundle By Name(cluster=T7 {"时间"=timestamp(0 s since 1904-01-01), "参数"="", "元器件"="", "故障现象"="", "故障分析"="", "state"="", "code"="", "platform_alarm_code"=""} ("data"), "时间"=w357, "参数"="CODMn", "元器件"=w356) -> (w354:T7)
                          n124 = call "挥发酚报警信息.vi"("data"=w354) -> ()  [unwired: 10 in, 1 out]
                        }
                      }
                    }
                  }
                  n125 = global write "VAR挥发酚全局变量.vi" "校准结果指示"(w286) -> ()
                }
              }
            }
          }
          frame #1 {
            n126 = call "校准数据写入配置文件.vi"() -> ()  [unwired: 11 in, 1 out]
          }
        }
      }
      frame "结束" {
        n127 = Release Queue(queue=w367) -> ()  [unwired: 2 in, 3 out]
        n128 = Release Notifier(notifier=w366) -> ()  [unwired: 2 in, 3 out]
      }
    }
    n129 = Not(x=w16) -> (.not. x?=w17:bool)
    n130 = global write "VAR挥发酚全局变量.vi" "校准任务"(w14) -> ()
    n131 = global write "VAR挥发酚全局变量.vi" "校准过程"(w12) -> ()
    n132 = global write "VAR挥发酚全局变量.vi" "校准运行状态"(w17) -> ()
  }
